vi "Data_to_CTD.vi"(1 "Data":T1) -> (0 "CommonTargetData":T2)   [LabVIEW 2011]
uses:
  CommonTargetData.ctl
  TargetData.ctl
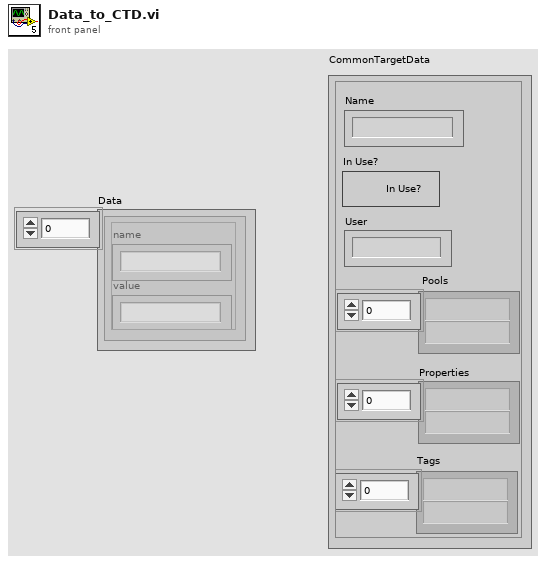
[diagram p1: front panel]
types:
  T1 = typedef "TargetData.ctl" = cluster{"name":string, "value":string}[]
  T2 = typedef "CommonTargetData.ctl" = cluster{"Name":string, "In Use?":bool, "User":string, " Pools":string[], "Tags":string[], "Properties":string[]}
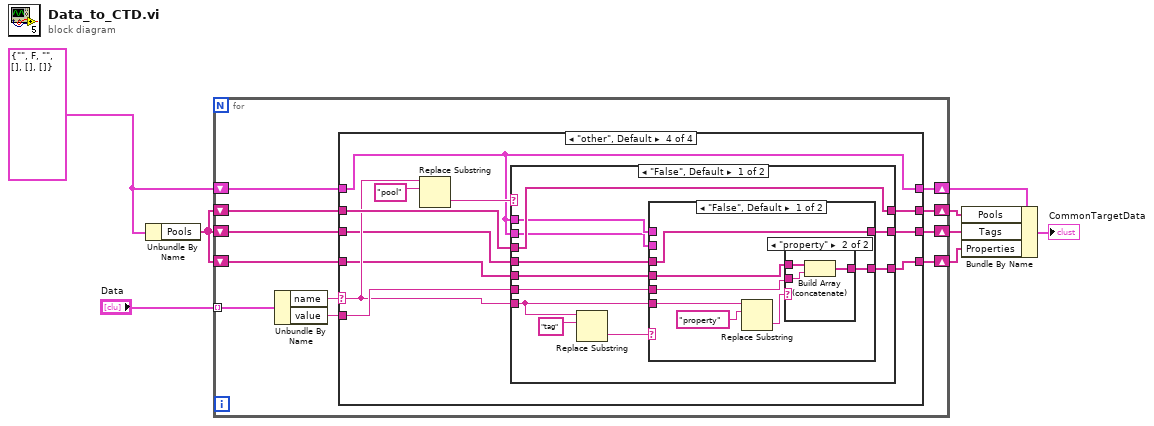
[diagram p0: block diagram]
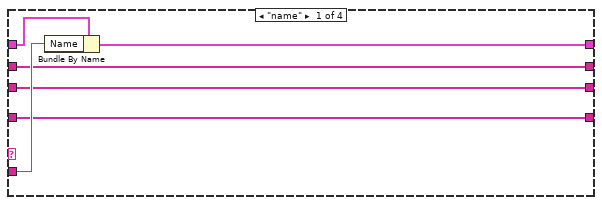
[diagram p2: hidden frame]
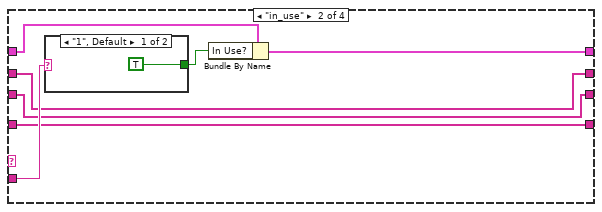
[diagram p3: hidden frame]
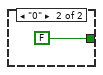
[diagram p4: hidden frame]
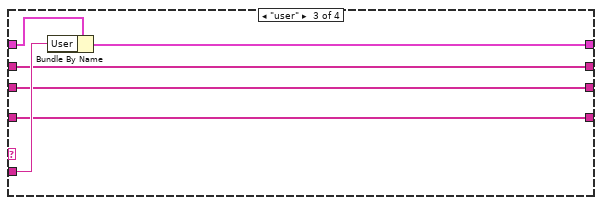
[diagram p5: hidden frame]
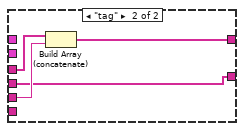
[diagram p7: hidden frame]
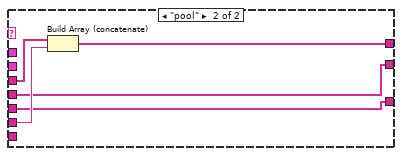
[diagram p8: hidden frame]
diagram:
  w1 = T2 {"Name"="", "In Use?"=FALSE, "User"="", " Pools"=[], "Tags"=[], "Properties"=[]} ("output cluster")
  n1 = Unbundle By Name(w1) -> ("Pools"=w4:string[])
  n2 = for {
    shift-right: [w16] -> w8
    shift-left: w1 -> [w17]
    shift-right: [w12] -> w5
    shift-left: w4 -> [w14]
    shift-right: [w13] -> w6
    shift-left: w4 -> [w15]
    shift-right: [w10] -> w3
    shift-left: w4 -> [w11]
    tunnel: "Data" -> [w9] mode=indexing
    n3 = Unbundle By Name(w9) -> ("name"=w19:string, "value"=w18:string)
    n4 = case shown="\"other\", Default" w19 {
      selector: w19 -> [_ _ _ w47]
      tunnel: w18 -> [w23 w30 w38 w49]
      tunnel: w17 -> [w25 w32 w40 w43]
      tunnel: [w24 w31 w39 w43] -> w16
      tunnel: w15 -> [w22 w27 w36 w51]
      tunnel: w14 -> [w21 w28 w37 w45]
      tunnel: [w22 w27 w36 w50] -> w13
      tunnel: [w21 w28 w37 w44] -> w12
      tunnel: w11 -> [w20 w26 w35 w42]
      tunnel: [w20 w26 w35 w41] -> w10
      frame "name" {
        n5 = Bundle By Name(cluster=w25, "Name"=w23) -> (w24:T2)
      }
      frame "in_use" {
        n6 = case shown="\"1\", Default" w30 {
          tunnel: [TRUE ("In Use?") FALSE ("In Use?")] -> w29
          frame "1", Default {
          }
          frame "0" {
          }
        }
        n7 = Bundle By Name(cluster=w32, "In Use?"=w29) -> (w31:T2)
      }
      frame "user" {
        n8 = Bundle By Name(cluster=w40, "User"=w38) -> (w39:T2)
      }
      frame "other", Default {
        n9 = Replace Substring(4:"pool" ("substring (\"\")"), 5:w47) -> (0:w46:string)  [unwired: 2 in, 1 out]
        n10 = case shown="\"False\", Default" w46 {
          tunnel: w51 -> [w62 w82]
          tunnel: [w62 w81] -> w50
          tunnel: w49 -> [w59 w80]
          tunnel: w47 -> [w55 _]
          tunnel: w45 -> [w58 w79]
          tunnel: [w57 w79] -> w44
          tunnel: w43 -> [w56 _]
          tunnel: w43 -> [w54 _]
          tunnel: w42 -> [w53 w78]
          tunnel: [w52 w78] -> w41
          frame "False", Default {
            n11 = Replace Substring(4:"tag" ("substring (\"\")"), 5:w55) -> (0:w60:string)  [unwired: 2 in, 1 out]
            n12 = case shown="\"False\", Default" w60 {
              tunnel: w59 -> [w64 w76]
              tunnel: w58 -> [w69 w77]
              tunnel: [w69 w75] -> w57
              tunnel: w56 -> [_ _]
              tunnel: w55 -> [w65 _]
              tunnel: w54 -> [_ _]
              tunnel: w53 -> [w66 w74]
              tunnel: [w63 w74] -> w52
              frame "False", Default {
                n13 = Replace Substring(4:"property" ("substring (\"\")"), 5:w65) -> (0:w67:string)  [unwired: 2 in, 1 out]
                n14 = case shown="\"property\"" w67 {
                  tunnel: w66 -> [w70 w73]
                  tunnel: w64 -> [_ w72]
                  tunnel: [w70 w71] -> w63
                  frame "False", Default {
                  }
                  frame "property" {
                    n15 = Build Array (concatenate)(w73, w72) -> (w71:string[])
                  }
                }
              }
              frame "tag" {
                n16 = Build Array (concatenate)(w77, w76) -> (w75:string[])
              }
            }
          }
          frame "pool" {
            n17 = Build Array (concatenate)(w82, w80) -> (w81:string[])
          }
        }
      }
    }
  }
  n18 = Bundle By Name(cluster=w8, "Pools"=w6, "Tags"=w5, "Properties"=w3) -> (→"CommonTargetData":T2)
